vi "Get SMO Serial Number.vi"(8 "error in (no error)":errorcluster, 11 "Inst.FP in":refnum<class "Inst.FP.lvclass">) -> (0 "error out":errorcluster, 2 "Serial Number":string, 3 "Inst.FP out":refnum<class "Inst.FP.lvclass">)   [LabVIEW 2019, in "Inst.FP.lvclass"]
doc: "Override this VI to return the serial number of your Instrument"
uses:
  Inst.FP.lvclass
  <userlib>/LevyLab/Instrument Framework/Instrument Types/Cryostat/Instrument.Cryostat.lvclass
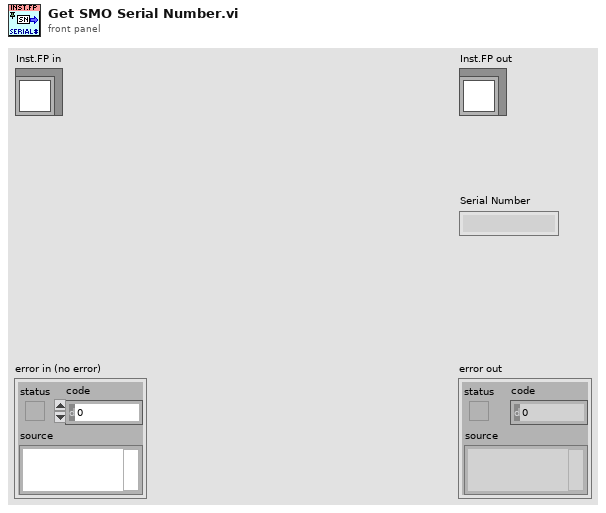
[diagram p1: front panel]
types:
  T1 = typedef "Inst.FP.lvclass/Inst.FP.Type--Enum.ctl" = enum32{"Wet", "CF"}
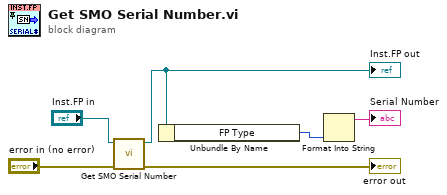
[diagram p0: block diagram]
diagram:
  n1 = call-parent "Get SMO Serial Number.vi"("error in (no error)"="error in (no error)", "Instrument in"="Inst.FP in") -> ("error out"=→"error out":errorcluster, "Instrument out"=w3:refnum<class "Inst.FP.lvclass">)  [unwired: 7 in, 1 out]
  "Inst.FP out" <- w3
  n2 = Unbundle By Name(w3) -> ("FP Type"=w2:T1)
  n3 = Format Into String(w2) -> (resulting string=→"Serial Number":string)  [unwired: 3 in, 1 out]
